vi "create.vi"(8 "error in (no error)":errorcluster) -> (0 "error out":errorcluster, 3 "CategoryList out":refnum<class "CategoryList.lvclass">)   [LabVIEW 2018, in "CategoryList.lvclass"]
uses:
  CategoryList.lvclass
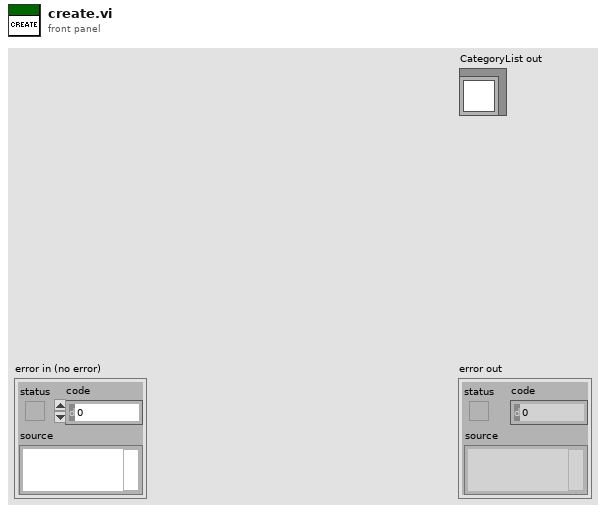
[diagram p1: front panel]
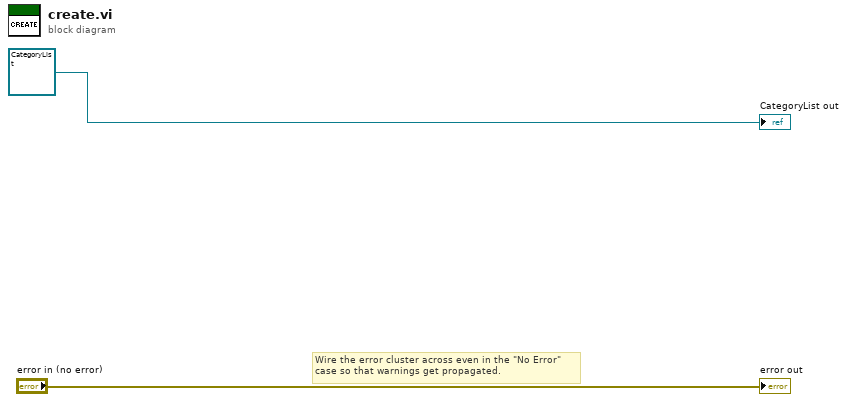
[diagram p0: block diagram]
diagram:
  # "Wire the error cluster across even in the \"No Error\"\ncase so that warnings get propagated."
  "error out" <- "error in (no error)"
  "CategoryList out" <- refnum<class "CategoryList.lvclass"> refnum ("CategoryList in")
